vi "Get File For Save.vi"(8 "error in (no error)":errorcluster caption="entrée d'erreur (pas d'erreur)", 11 "Class Instrument Log_File en entrée":refnum<class "Class Instrument Log_File.lvclass">) -> (0 "error out":errorcluster caption="sortie d'erreur", 2 "File For Save":refnum<queue>, 3 "Class Instrument Log_File en sortie":refnum<class "Class Instrument Log_File.lvclass">)   [LabVIEW 2020, in "Library Instrument & Equipement.lvlib" / "Library Instruments.lvlib" / "Class Instrument Log_File.lvclass"]
uses:
  Class Instrument Log_File.lvclass
  Commun VI/TypeDef/Commande Test/Commande Data Test.ctl
  Commun VI/TypeDef/Commande Test/Commande Value Type.ctl
  Commun VI/TypeDef/Commande Test/Commande Type Test.ctl
  Class Instrument Log_File.lvclass/Class Instrument Log_File.ctl
  Commun VI/Library Commun.lvlib
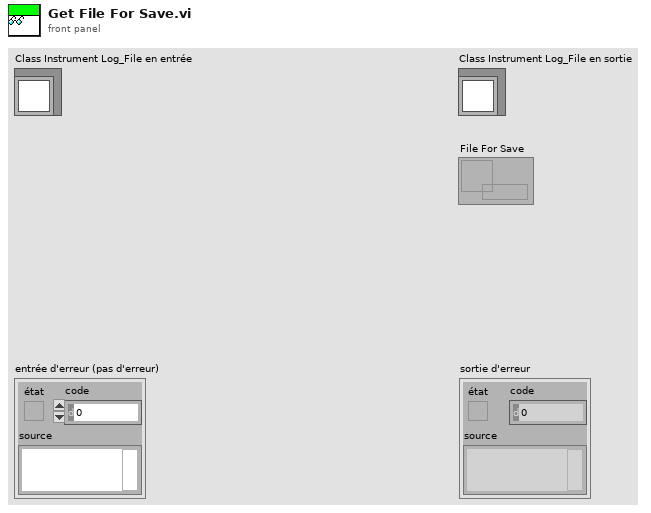
[diagram p1: front panel]
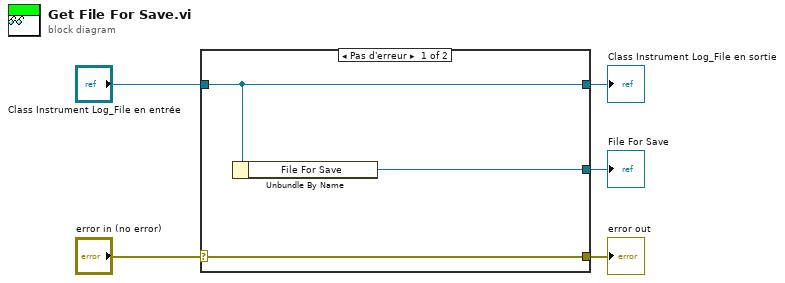
[diagram p0: block diagram]
diagram:
  n1 = case shown="Pas d'erreur" "error in (no error)" {
    selector: "error in (no error)" -> [w8 w9]
    tunnel: [w8 w9] -> w4
    tunnel: [w7 w10] -> w2
    tunnel: "Class Instrument Log_File en entrée" -> [w7 w10]
    tunnel: [w6 _] -> w1
    frame No Error {
      n2 = Unbundle By Name(w7) -> ("File For Save"=w6:refnum<queue>)
    }
    frame Error {
    }
  }
  "error out" <- w4
  "Class Instrument Log_File en sortie" <- w2
  "File For Save" <- w1
